vi "Get Mediator Message.vi"(8 "error in (no error)":errorcluster, 11 "Message AF Mediator in":refnum<class "Message AF Mediator.lvclass">) -> (0 "error out":errorcluster, 2 "Mediator Message":refnum<class "Message Interface.lvclass">, 3 "Message AF Mediator out":refnum<class "Message AF Mediator.lvclass">)   [LabVIEW 2016, in "Stream Mediator.lvlib" / "Message AF Mediator.lvclass"]
doc: "--\nCopyright © 2017 Composed SystemsI All rights reserved.\n\nAuthor: Jon McBee <jon.mcbee@composed.io>\n\nThis library is provided \"AS IS\" ,WITHOUT WARRANTIES OR\nCONDITIONS OF ANY KIND, either express or implied.\n\nComposed Systems -- composed.io\n\nStream 0.0.1.1\nJon McBee - Composed Systems\nCopyright (c) 2017, Composed Systems"
uses:
  <userlib>/Composed Systems/Stream/Mediator/Classes/Message AF Mediator/Message AF Mediator.lvclass
  <userlib>/Composed Systems/Stream/Mediator/Classes/Message Interface/Message Interface.lvclass
  <userlib>/Composed Systems/Stream/Mediator/Classes/Message AF Mediator/Message AF Mediator.lvclass/Message AF Mediator.ctl
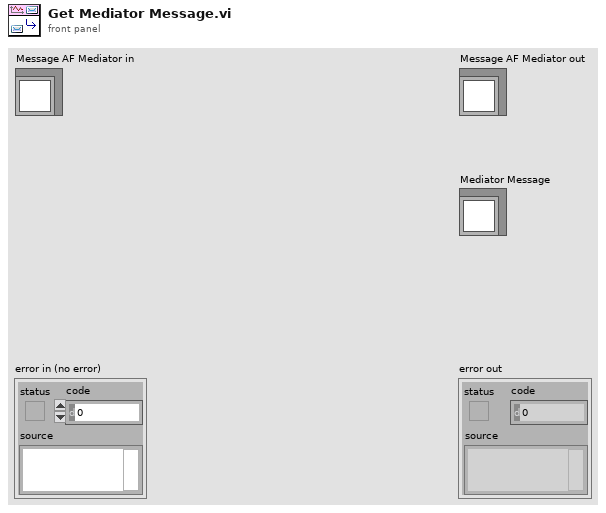
[diagram p1: front panel]
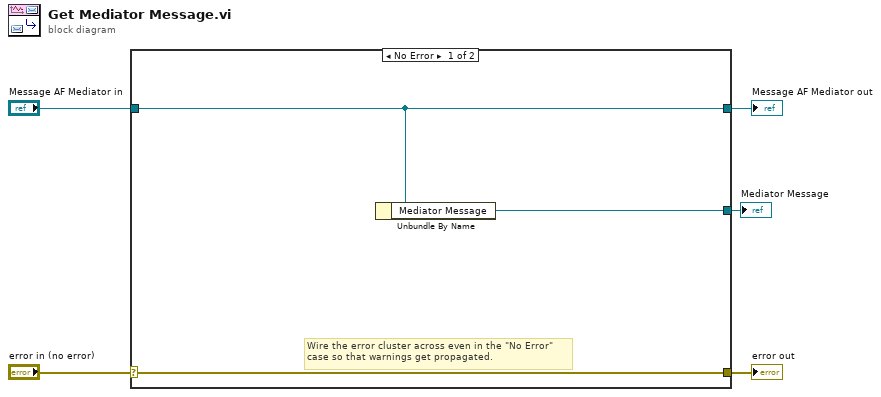
[diagram p0: block diagram]
diagram:
  n1 = case shown="No Error" "error in (no error)" {
    selector: "error in (no error)" -> [w8 w10]
    tunnel: [w8 w10] -> w4
    tunnel: [w7 w9] -> w2
    tunnel: "Message AF Mediator in" -> [w7 w9]
    tunnel: [w6 _] -> w1
    frame No Error {
      # "Wire the error cluster across even in the \"No Error\"\ncase so that warnings get propagated."
      n2 = Unbundle By Name(w7) -> ("Mediator Message"=w6:refnum<class "Message Interface.lvclass">)
    }
    frame Error {
    }
  }
  "error out" <- w4
  "Message AF Mediator out" <- w2
  "Mediator Message" <- w1
